vi "ZDataVIS_get_processed_directory.vi"(10 "increment (T) or overwrite (F) folders":bool, 11 "File Information":T1={"File or folder path (input)"=path "G:/My Drive/ansom/Data/PPMS2/SA03008L.20190612/004_SG_IV_Testing", "output file description"="yonk"}) -> (3 "root processed directory":path)   [LabVIEW 2016]
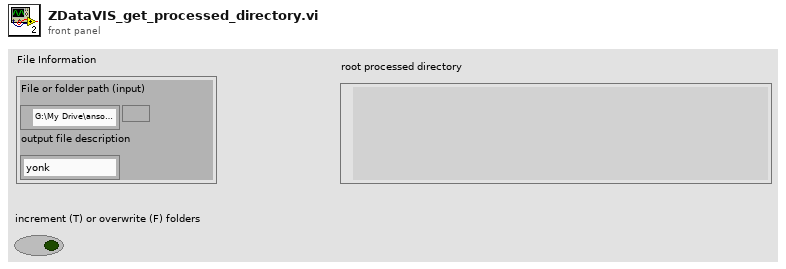
[diagram p1: front panel]
types:
  T1 = cluster{"File or folder path (input)":path, "output file description":string}
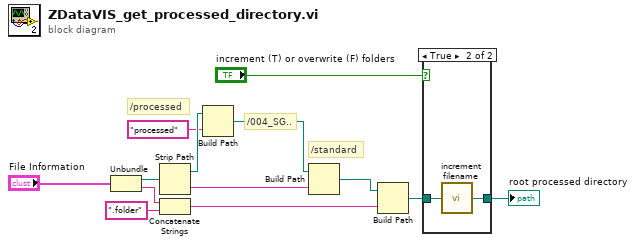
[diagram p0: block diagram]
diagram:
  # "/standard"
  # "/004_SG.."
  # "/processed"
  n1 = Unbundle("File Information") -> ("File or folder path (input)"=w2:path, "output file description"=w1:string)
  n2 = Strip Path(path=w2) -> (stripped path=w13:path, name=w10:string)
  n3 = Concatenate Strings(w1, ".folder" ("string")) -> (w7:string)
  n4 = Build Path(base path=w13, name or relative path="processed") -> (appended path=w11:path)
  n5 = Build Path(base path=w11, name or relative path=w10) -> (appended path=w9:path)
  n6 = Build Path(base path=w9, name or relative path=w7) -> (appended path=w8:path)
  n7 = case shown="True" "increment (T) or overwrite (F) folders" {
    tunnel: w8 -> [w14 w16]
    tunnel: [w14 w15] -> w4
    frame False {
    }
    frame True {
      n8 = call <userlib>:"increment filename.vi"("path"=w16) -> ("modified path"=w15:path)
    }
  }
  "root processed directory" <- w4
